vi "Target_FIFO_ZERO.vi"() -> ()   [LabVIEW 2018]
uses:
  <vilib>/rvi/Emulation/niFpgaGetClockAttributes.vi
  <vilib>/rvi/Emulation/niFpgaSctlEmulationGetInTimedLoop.vi
  <vilib>/rvi/Emulation/niFpgaEmulationReportErrorSimple.vi
  <vilib>/rvi/interface/RandomDataEmulation/niFpgaRandomDataHandleErrors.vi
  <vilib>/rvi/Emulation/niFpgaCriticalErrorInLSC.vi
  <vilib>/rvi/DataTransferAndStorage/Container/XNode/niFpgaContainer.xnode
  <vilib>/rvi/interface/RandomDataEmulation/nirviRandomDataFpgaReadWriteTemplate.vi
panel:
  in  "Timeout":i32
  out "Number of Elements to Write":u32
  in  "Сколько в ФИФО?":bool
  in  "Element":u8
  in  "Запись в ФИФО":bool
  in  "Count(mSec)":u32
  in  "stop":bool
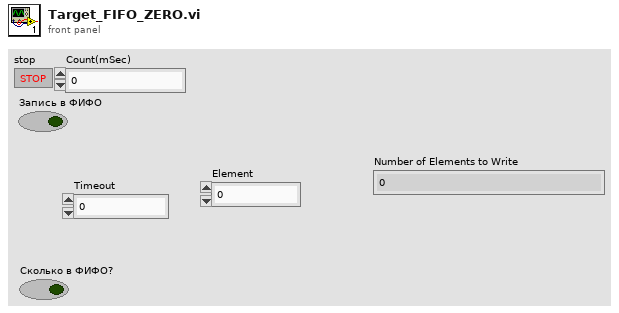
[diagram p1: front panel]
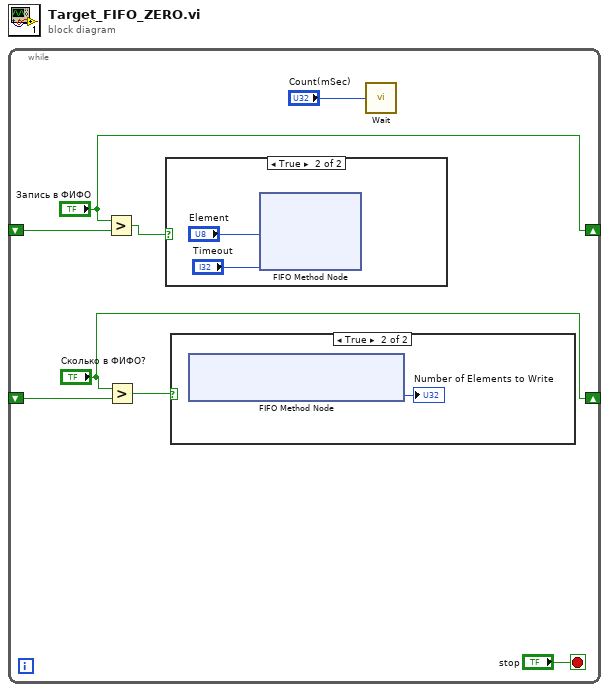
[diagram p0: block diagram]
diagram:
  n1 = while {
    shift-right: ["Запись в ФИФО"] -> _
    shift-left: _ -> [w6]
    shift-right: ["Сколько в ФИФО?"] -> _
    shift-left: _ -> [w3]
    stop <- "stop" stop-if-true
    n2 = Greater?(x="Запись в ФИФО", y=w6) -> (0:w4:bool)
    n3 = Greater?(x="Сколько в ФИФО?", y=w3) -> (0:w2:bool)
    n4 = case shown="True" w4 {
      frame False {
      }
      frame True {
        n5 = xnode ("FIFO Method Node")("Element"="Element", "Timeout"="Timeout") -> ()  [unwired: 1 in, 2 out]
      }
    }
    n6 = case shown="True" w2 {
      frame False {
      }
      frame True {
        n7 = xnode ("FIFO Method Node")() -> ("Number of Elements to Write"=→"Number of Elements to Write":u32)  [unwired: 1 in, 1 out]
      }
    }
    n8 = call "Wait"("Count(mSec)"="Count(mSec)") -> ()  [unwired: 1 out]
  }
